vi "JWT Elements.vi"(7 "Client ID":string, 8 "error in (no error)":errorcluster, 10 "id_token":string, 11 "JSONWebToken in":refnum<class "JSONWebToken.lvclass">) -> (0 "error out":errorcluster, 3 "JSONWebToken out":refnum<class "JSONWebToken.lvclass">)   [LabVIEW 2017, in "JSONWebToken.lvclass"]
doc: "Parses the JWT parts for access via private data"
uses:
  JSONWebToken.lvclass
  JSONWebToken.lvclass/JSONWebToken.ctl
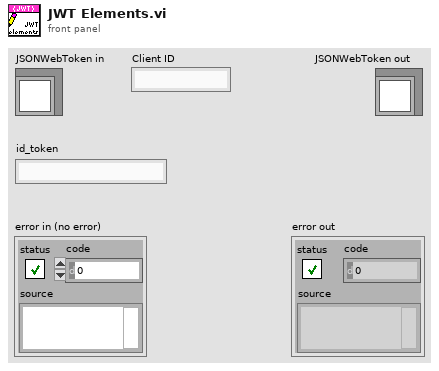
[diagram p1: front panel]
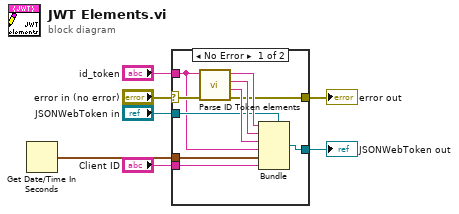
[diagram p0: block diagram]
diagram:
  n1 = Get Date/Time In Seconds() -> (seconds since 1Jan1904=w2:timestamp)
  n2 = case shown="No Error" "error in (no error)" {
    selector: "error in (no error)" -> [w14 w18]
    tunnel: [w13 w18] -> w6
    tunnel: [w11 w19] -> w4
    tunnel: "JSONWebToken in" -> [w12 w19]
    tunnel: "id_token" -> [w10 _]
    tunnel: w2 -> [w9 _]
    tunnel: "Client ID" -> [w8 _]
    frame No Error {
      n3 = call "Parse ID Token elements.vi"("error in (no error)"=w14, "ID Token"=w10) -> ("error out"=w13:errorcluster, "signature"=w17:string, "payload"=w15:string, "header"=w16:string)  [unwired: 6 in]
      n4 = Bundle(cluster=w12, w16, w15, w17, w10, w9, w8) -> (w11:refnum<class "JSONWebToken.lvclass">)
    }
    frame Error {
    }
  }
  "error out" <- w6
  "JSONWebToken out" <- w4
